vi "Get ID.vi"(8 "error in (no error)":errorcluster, 10 "name":string, 11 "Formatting Handler in":refnum<class "Formatting Handler.lvclass">) -> (0 "error out":errorcluster, 2 "ID":i32, 3 "Formatting Handler out":refnum<class "Formatting Handler.lvclass">)   [LabVIEW 2018, in "GLog.lvlib" / "Formatting Handler.lvclass"]
uses:
  Formatting Handler.lvclass
panel:
  # "Connector Pane"
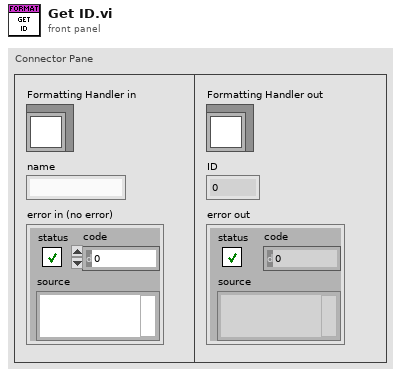
[diagram p1: front panel]
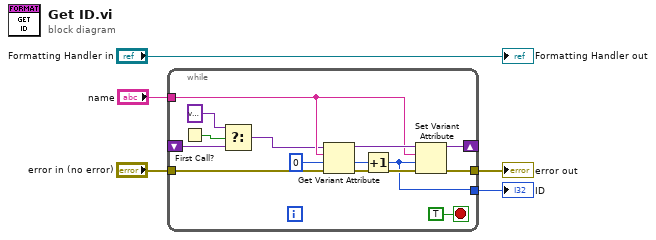
[diagram p0: block diagram]
diagram:
  n1 = while {
    shift-right: [w17] -> _
    shift-left: _ -> [w7]
    tunnel: "name" -> [w15]
    tunnel: "error in (no error)" -> [w13]
    tunnel: [w12] -> w2
    tunnel: [w11] -> w1
    stop <- TRUE stop-if-true
    n2 = First Call?() -> (First Call?: T/F=w9:bool)
    n3 = Select(t=variant, s=w9, f=w7) -> (s? t:f=w6:variant)
    n4 = Get Variant Attribute(Variant=w6, name=w15, default value (empty Variant)=0, error in=w13) -> (duplicate Variant=w18:variant, value=w16:i32, error out=w14:errorcluster)  [unwired: 1 out]
    n5 = Increment(x=w16) -> (x+1=w11:i32)
    n6 = Set Variant Attribute(Variant=w18, name=w15, value=w11, error in=w14) -> (Variant out=w17:variant, error out=w12:errorcluster)  [unwired: 1 out]
  }
  "error out" <- w2
  "ID" <- w1
  "Formatting Handler out" <- "Formatting Handler in"
